vi "GotoWaypoint.vi"(7 "InhibitIn":bool, 8 "CurrentSteerAngle":dbl, 9 "WhatAroundMe? Clean":cluster{"T":dbl, "Range":dbl, "Bearing":dbl}[](array[cluster]), 10 "WhereAmI? Clean":T3, 11 "MDF In":T2(array[cluster])) -> (0 "BehCom":T1(ring), 1 "MDF Out":T2(array[cluster]), 2 "ActCommand":dbl[](array[numeric]), 4 "InhibitOut":bool, 5 "Vel":dbl, 6 "SteerAngle":dbl)   [LabVIEW 2012]
doc: "This subVI contains the Forebrain Goto Waypoint behaviors. Its inputs are the outputs of thewhat and where SENSE processes, theMission efinition Filet, a suppression value from another co-brahvior and an inhibit signal to turn the behavior off. The outputs are a 90 element steering array and a suppression value to diminish the output of co-behaviors.\n\nIt is designed to work with a 90 element behavior arbiter."
uses:
  <vilib>/Analysis/1siggen.llb/Ramp Pattern by Samples.vi
  <vilib>/gmath/statdist.llb/Normal PDF.vi
  <vilib>/gmath/NI_Gmath.lvlib
  <vilib>/Analysis/NI_AALBase.lvlib
panel:
  out "loop index":i32
  in  "HowAmI? Clean":cluster{"T":dbl, "Battery":dbl, "Temp":dbl}
  # "This VI contains the go to waypoint behavior  at the Forebrain level"
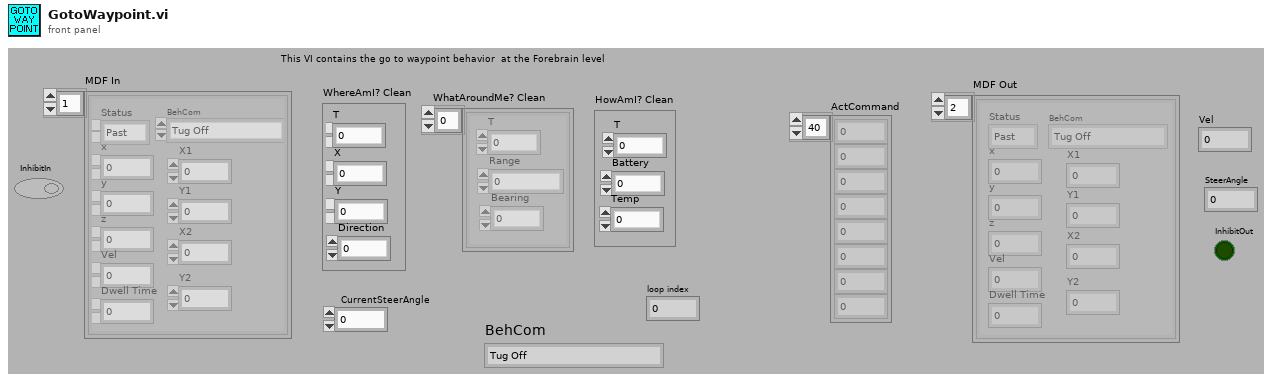
[diagram p1: front panel]
types:
  T1 = enum16{"Tug Off", "Manual Mode", "Goto WayPoint", "Back Up", "Circle", "Left Wall Follow", "Right Wall Follow", "Hunt"}
  T2 = cluster{"Status":enum16{"Past", "Current", "Future"}, "x":dbl, "y":dbl, "z":dbl, "Vel":dbl, "Dwell Time":dbl, "BehCom":enum16{"Tug Off", "Manual Mode", "Goto WayPoint", "Back Up", "Gate", "Left Wall Follow", "Right Wall Follow", "Hunt"}, "X1":dbl, "Y1":dbl, "X2":dbl, "Y2":dbl}[]
  T3 = cluster{"T":dbl, "X":dbl, "Y":dbl, "Direction":dbl}
  T4 = enum16{"Tug Off", "Manual Mode", "Goto WayPoint", "Back Up", "Gate", "Left Wall Follow", "Right Wall Follow", "Hunt"}
  T5 = cluster{"Status":enum16{"Past", "Current", "Future"}, "x":dbl, "y":dbl, "z":dbl, "Vel":dbl, "Dwell Time":dbl, "BehCom":enum16{"Tug Off", "Manual Mode", "Goto WayPoint", "Back Up", "Gate", "Left Wall Follow", "Right Wall Follow", "Hunt"}, "X1":dbl, "Y1":dbl, "X2":dbl, "Y2":dbl}
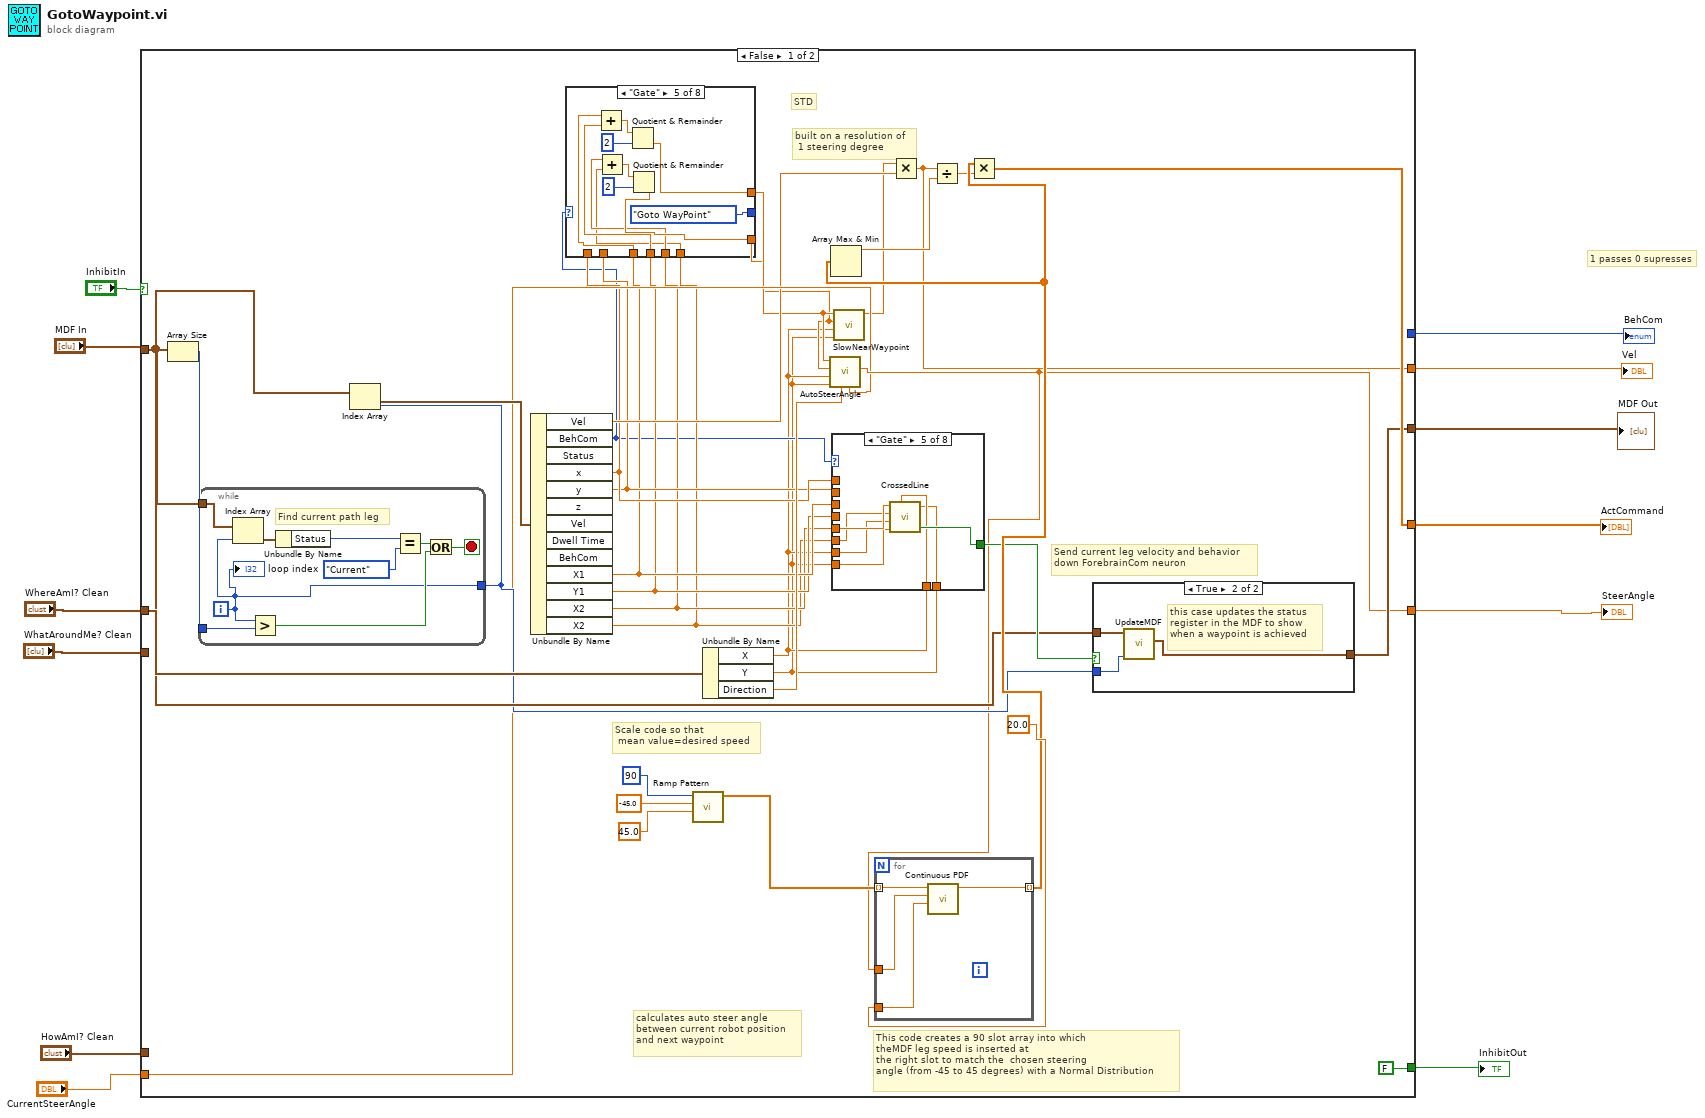
[diagram p0: block diagram]
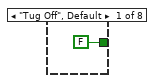
[diagram p9: hidden frame]
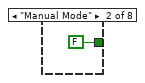
[diagram p10: hidden frame]
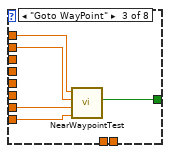
[diagram p11: hidden frame]
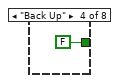
[diagram p12: hidden frame]
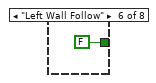
[diagram p13: hidden frame]
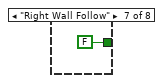
[diagram p14: hidden frame]
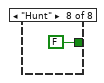
[diagram p15: hidden frame]
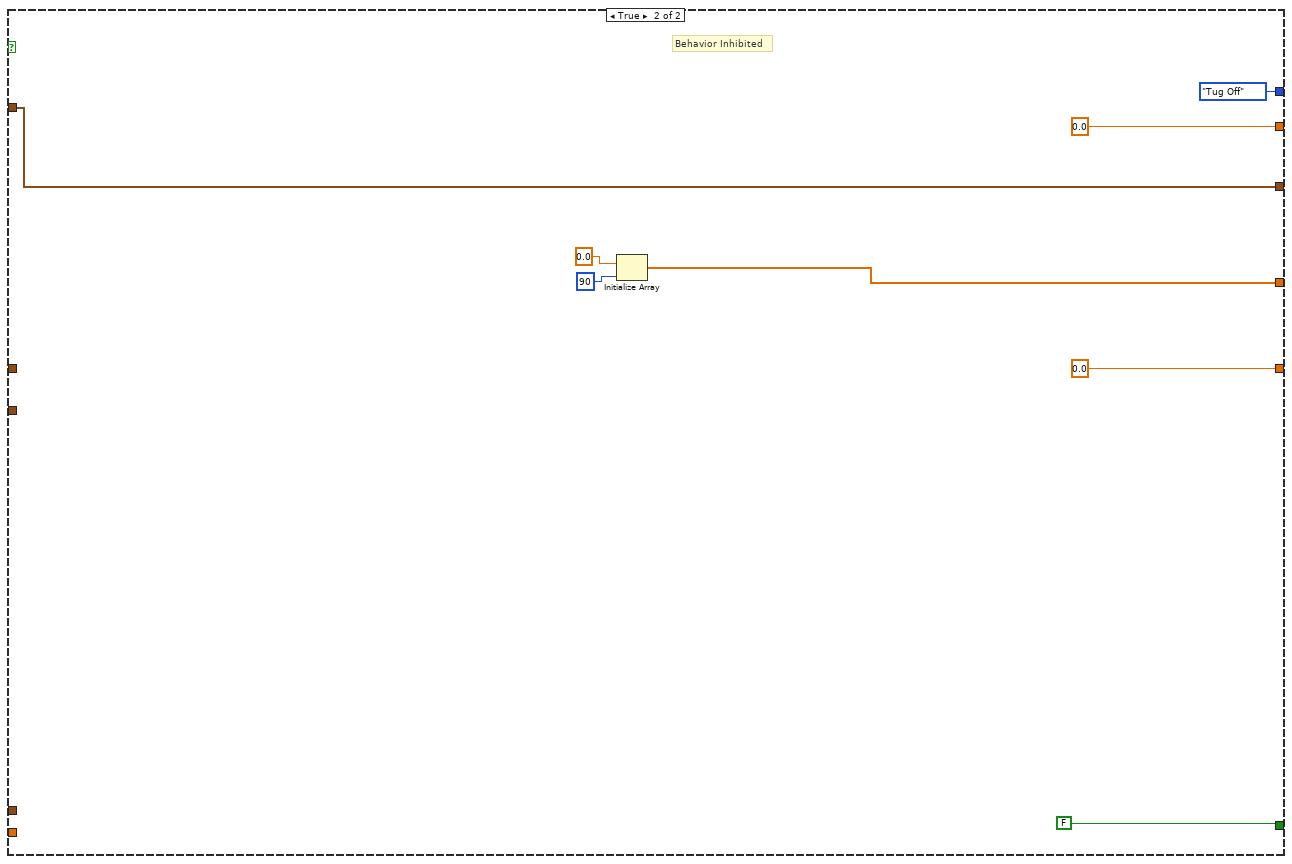
[diagram p17: hidden frame]
diagram:
  # "1 passes 0 supresses"
  n1 = case shown="False" "InhibitIn" {
    tunnel: "WhatAroundMe? Clean" -> [_ _]
    tunnel: "WhereAmI? Clean" -> [w44 _]
    tunnel: "HowAmI? Clean" -> [_ _]
    tunnel: [w34 w120] -> w8
    tunnel: [FALSE ("InhibitOut") FALSE ("InhibitOut")] -> w1
    tunnel: "MDF In" -> [w31 w117]
    tunnel: [w30 w117] -> w6
    tunnel: [w25 0.0 ("Vel")] -> w5
    tunnel: [w28 0.0 ("SteerAngle")] -> w4
    tunnel: "CurrentSteerAngle" -> [w27 _]
    tunnel: [_ T1."Tug Off" ("BehCom")] -> w2
    frame False {
      # "Send current leg velocity and behavior\ndown ForebrainCom neuron"
      # "calculates auto steer angle\nbetween current robot position\nand next waypoint"
      # "built on a resolution of\n 1 steering degree"
      # "Scale code so that\n mean value=desired speed"
      # "STD"
      # "This code creates a 90 slot array into which\ntheMDF leg speed is inserted at\nthe right slot to match the  chosen steering\nangle (from -45 to 45 degrees) with a Normal Distribution"
      n2 = Array Size(array=w31) -> (size(s)=w45:i32)
      n3 = while {
        tunnel: w45 -> [w113]
        tunnel: w31 -> [w110]
        tunnel: [w105] -> w29
        i -> [w105]
        stop <- w112 stop-if-true
        # "Find current path leg"
        n4 = Index Array "Index Array"(array=w110, index=w105) -> (element=w107:T5)
        n5 = Greater?(x=w105, y=w113) -> (0:w111:bool)
        n6 = Unbundle By Name(w107) -> ("Status"=w108:enum16{"Past", "Current", "Future"})
        n7 = Equal?(x=w108, y=enum16{"Past", "Current", "Future"}."Current") -> (x = y?=w109:bool)
        n8 = Or(x=w109, y=w111) -> (x .or. y?=w112:bool)
        "loop index" <- w105
      }
      n9 = Index Array "Index Array"(array=w31, index=w29) -> (element=w43:T5)
      n10 = Unbundle By Name(w43) -> ("Vel"=w26:dbl, "BehCom"=w17:T4, "x"=w23:dbl, "y"=w22:dbl, "X1"=w21:dbl, "Y1"=w20:dbl, "X2"=w19:dbl, "X2"=w18:dbl)  [unwired: 5 out]
      n11 = case shown="\"Gate\"" w17 {
        selector: w17 -> [w49 w52 w55 w58 _ w72 w75 w78]
        tunnel: [w49 w52 w55 w58 T4."Goto WayPoint" ("BehCom") w72 w75 w78] -> _
        tunnel: w23 -> [w47 w50 w54 w56 _ w71 w73 w76]
        tunnel: w22 -> [w48 w51 w53 w57 _ w70 w74 w77]
        tunnel: w21 -> [_ _ _ _ w66 _ _ _]
        tunnel: w20 -> [_ _ _ _ w65 _ _ _]
        tunnel: w19 -> [_ _ _ _ w64 _ _ _]
        tunnel: w18 -> [_ _ _ _ w63 _ _ _]
        tunnel: [w48 w51 w53 w57 w68 w70 w74 w77] -> w15
        tunnel: [w47 w50 w54 w56 w67 w71 w73 w76] -> w16
        frame "Tug Off", Default {
        }
        frame "Manual Mode" {
        }
        frame "Goto WayPoint" {
        }
        frame "Back Up" {
        }
        frame "Gate" {
          n12 = Add(x=w66, y=w65) -> (x+y=w61:dbl)
          n13 = Add(x=w64, y=w63) -> (x+y=w62:dbl)
          n14 = Quotient & Remainder(x=w61, y=2) -> (floor(x/y)=w67:dbl)  [unwired: 1 out]
          n15 = Quotient & Remainder(x=w62, y=2) -> (floor(x/y)=w68:dbl)  [unwired: 1 out]
        }
        frame "Left Wall Follow" {
        }
        frame "Right Wall Follow" {
        }
        frame "Hunt" {
        }
      }
      n16 = call-poly <vilib>:"Ramp Pattern.vi"("start"=45.0, "end"=-45.0 ("end (Normal)"), "samples"=90) -> ("Ramp Pattern"=w37:dbl[])  [unwired: 7 in, 1 out]
      n17 = Unbundle By Name(w44) -> ("X"=w14:dbl, "Y"=w13:dbl, "Direction"=w33:dbl)
      n18 = call "AutoSteerAngle.vi"("CurrentSteerAngle"=w27, "CurrentDirection"=w33, "Ycurrent"=w13, "Xcurrent"=w14, "Ywaypoint"=w15, "Xwaypoint"=w16) -> ("NewSteerAngle"=w28:dbl)  [unwired: 5 in]
      n19 = case shown="\"Gate\"" w17 {
        tunnel: [FALSE FALSE w85 FALSE w93 FALSE FALSE FALSE] -> w32
        tunnel: w23 -> [_ _ w84 _ _ _ _ _]
        tunnel: w22 -> [_ _ w83 _ _ _ _ _]
        tunnel: w14 -> [_ _ w82 _ w90 _ _ _]
        tunnel: w13 -> [_ _ w81 _ w89 _ _ _]
        tunnel: w21 -> [_ _ _ _ _ _ _ _]
        tunnel: w20 -> [_ _ _ _ _ _ _ _]
        tunnel: w19 -> [_ _ _ _ w92 _ _ _]
        tunnel: w18 -> [_ _ _ _ w91 _ _ _]
        tunnel: w14 -> [_ _ _ _ w88 _ _ _]
        tunnel: w13 -> [_ _ _ _ w87 _ _ _]
        frame "Tug Off", Default {
        }
        frame "Manual Mode" {
        }
        frame "Goto WayPoint" {
          n20 = call "NearWaypointTest.vi"("Yrobot"=w81, "Xrobot"=w82, "Ywaypoint"=w83, "Xwaypoiny"=w84) -> ("AtWaypoint"=w85:bool)  [unwired: 7 in]
        }
        frame "Back Up" {
        }
        frame "Gate" {
          n21 = call "CrossedLine.vi"("Xpoint1"=w92, "XpointC"=w88, "Ypoint1"=w91, "Xpoint2"=w90, "Ypoint2"=w89, "YpointC"=w87) -> ("CrossedLine"=w93:bool)  [unwired: 2 in]
        }
        frame "Left Wall Follow" {
        }
        frame "Right Wall Follow" {
        }
        frame "Hunt" {
        }
      }
      n22 = call "SlowNearWaypoint.vi"("Yrobot"=w13, "Xrobot"=w14, "Ywaypoint"=w15, "Xwaypoiny"=w16) -> ("SpeedDecrease"=w24:dbl)  [unwired: 7 in]
      n23 = for {
        tunnel: w37 -> [w104] mode=indexing
        tunnel: 20.0 ("std (Normal)") -> [w103]
        tunnel: [w102] -> w41 mode=indexing
        tunnel: w28 -> [w101]
        n24 = call-poly <vilib>:"Continuous PDF.vi"("std"=w103, "mean"=w101, "x"=w104) -> ("pdf(x)"=w102:dbl)  [unwired: 7 in, 1 out]
      }
      n25 = Array Max & Min(array=w41) -> (max value=w39:dbl)  [unwired: 3 out]
      n26 = Multiply(x=w24, y=w26) -> (x*y=w25:dbl)
      n27 = Divide(x=w25, y=w39) -> (x/y=w40:dbl)
      n28 = Multiply(x=w41, y=w40) -> (x*y=w34:dbl[])
      n29 = case shown="True" w32 {
        tunnel: w31 -> [w97 w100]
        tunnel: [w97 w98] -> w30
        tunnel: w29 -> [_ w99]
        frame False {
          # "robot not near waypoint\npass MDF through unaltered"
        }
        frame True {
          # "this case updates the status\nregister in the MDF to show \nwhen a waypoint is achieved"
          n30 = call "UpdateMDF.vi"("Index"=w99, "MDF_In"=w100) -> ("MDF_Out"=w98:T2)  [unwired: 9 in]
        }
      }
    }
    frame True {
      # "Behavior Inhibited"
      n31 = Initialize Array "Initialize Array"(0.0 ("element"), 90 ("dimension size")) -> (w120:dbl[])
    }
  }
  "ActCommand" <- w8
  "InhibitOut" <- w1
  "MDF Out" <- w6
  "Vel" <- w5
  "SteerAngle" <- w4
  "BehCom" <- w2
